vi "GOMDBTS2048 spectral Get Measurement Time Inus.vi"(8 "error in (no error)":errorcluster, 11 "handle":i32) -> (0 "error out":errorcluster, 2 "function return":i32, 3 "timeInus":i32)   [LabVIEW 2015, in "GOMDBTS2048.lvlib"]
doc: "GOBTS2048DLL int __stdcall GOMDBTS2048_spectralGetIntegrationTimeInus(int handle, int* timeInus);"
uses:
  GOMDBTS2048.lvlib
  runtime/GOMDBTS2048.dll
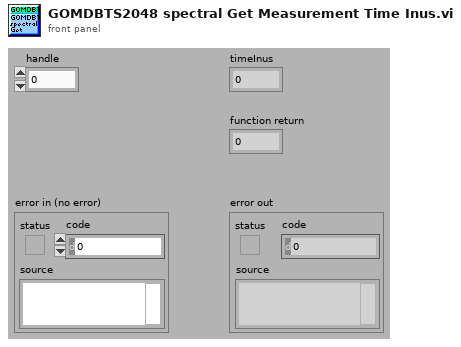
[diagram p1: front panel]
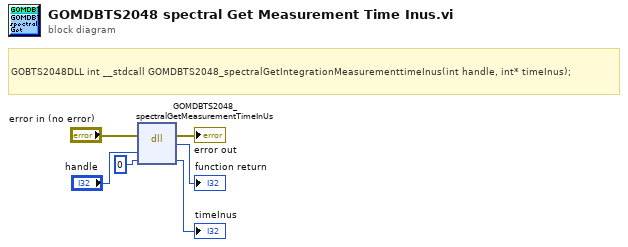
[diagram p0: block diagram]
diagram:
  # "GOBTS2048DLL int __stdcall GOMDBTS2048_spectralGetIntegrationMeasurementtimeInus(int handle, int* timeInus);"
  n1 = dll-call lib="C:/Users/rkoch/Documents/GO_Library/runtime/GOMDBTS2048.*" fn="GOMDBTS2048_spectralGetMeasurementTimeInUs"(error in="error in (no error)", "handle"="handle", "timeInus"=0) -> (error out=→"error out":errorcluster, "return type"=→"function return":i32, "timeInus"=→"timeInus":i32)  [unwired: 3 in, 1 out]
